vi "Graph MinMax X.vi"(8 "Fehler (Eingang, kein Fehler)":errorcluster, 10 "Max. Wert":dbl, 11 "Signalverlaufsdiagramm (Eingang)":refnum<vi>[](array[refnum])) -> (0 "Fehler (Ausgang)":errorcluster, 2 "Max. Wert out":dbl, 3 "Signalverlaufsdiagramm (Ausgang)":refnum<vi>[](array[refnum]))   [LabVIEW 2020, in "EPA 1065.lvlib" / "HovaCAL Interference verificaton.lvlib"]
uses:
  HovaCAL Interference verificaton.lvlib
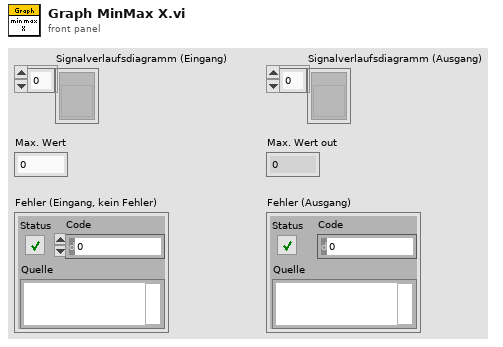
[diagram p1: front panel]
types:
  T1 = typedef "LVDateTimeRec.ctl" = cluster{"Sekundenbruchteil":dbl, "Sekunde":i32, "Minute":i32, "Stunde":i32, "Tag des Monats":i32, "Monat":i32, "Jahr":i32, "Wochentag":i32, "Tag des Jahres":i32, "DST":i32}
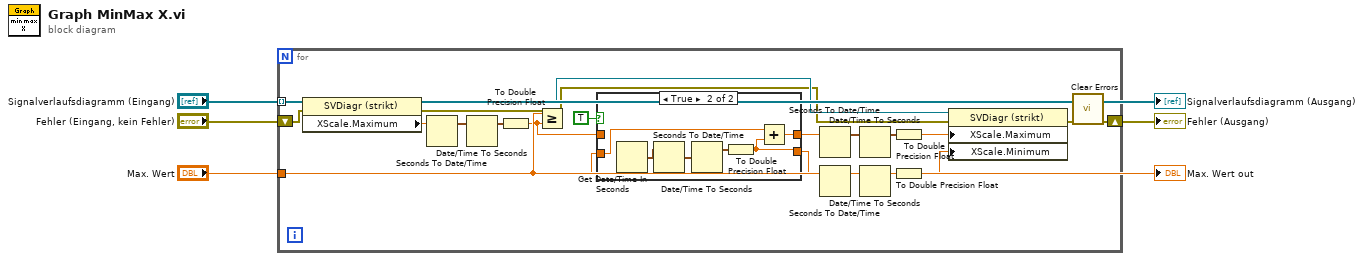
[diagram p0: block diagram]
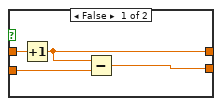
[diagram p2: hidden frame]
diagram:
  n1 = for {
    tunnel: "Max. Wert" -> [w23]
    tunnel: "Signalverlaufsdiagramm (Eingang)" -> [w22] mode=indexing
    shift-right: [w17] -> w2
    shift-left: "Fehler (Eingang, kein Fehler)" -> [w19]
    n2 = property on="Eigenschaftsknoten" class="SVDiagr (strikt)"(reference=w22, error in=w19) -> (reference out=w21:refnum<vi>, error out=w20:errorcluster, "XScale.Maximum"=w24:dbl)
    n3 = Seconds To Date/Time(time stamp (now)=w24) -> (date time rec=w16:T1)  [unwired: 1 in]
    n4 = Date/Time To Seconds(2:w16) -> (0:w14:timestamp)  [unwired: 1 in]
    n5 = To Double Precision Float(number=w14) -> (double precision float=w15:dbl)
    n6 = Greater Or Equal?(x=w23, y=w15) -> ()  [unwired: 1 out]
    n7 = case shown="True" TRUE ("x >= y?") {
      tunnel: w23 -> [w26 w34]
      tunnel: w15 -> [w28 _]
      tunnel: [w25 w30] -> w8
      tunnel: [w27 w29] -> w5
      frame False {
        n8 = Increment(x=w28) -> (x+1=w25:dbl)
        n9 = Subtract(x=w25, y=w26) -> (x-y=w27:dbl)
      }
      frame True {
        n10 = Get Date/Time In Seconds() -> (seconds since 1Jan1904=w32:timestamp)
        n11 = Seconds To Date/Time(time stamp (now)=w32) -> (date time rec=w31:T1)  [unwired: 1 in]
        n12 = Date/Time To Seconds(2:w31) -> (0:w33:timestamp)  [unwired: 1 in]
        n13 = To Double Precision Float(number=w33) -> (double precision float=w29:dbl)
        n14 = Add(x=w34, y=w29) -> (x+y=w30:dbl)
      }
    }
    n15 = Seconds To Date/Time(time stamp (now)=w8) -> (date time rec=w13:T1)  [unwired: 1 in]
    n16 = Seconds To Date/Time(time stamp (now)=w5) -> (date time rec=w9:T1)  [unwired: 1 in]
    n17 = Date/Time To Seconds(2:w13) -> (0:w12:timestamp)  [unwired: 1 in]
    n18 = Date/Time To Seconds(2:w9) -> (0:w10:timestamp)  [unwired: 1 in]
    n19 = To Double Precision Float(number=w12) -> (double precision float=w11:dbl)
    n20 = To Double Precision Float(number=w10) -> (double precision float=w7:dbl)
    n21 = property on="Eigenschaftsknoten" class="SVDiagr (strikt)"(reference=w21, error in=w20, "XScale.Maximum"=w11, "XScale.Minimum"=w7) -> (error out=w18:errorcluster)  [unwired: 1 out]
    n22 = call <vilib>:"Clear Errors.vi"("error in (no error)"=w18) -> ("error out"=w17:errorcluster)  [unwired: 5 in, 1 out]
  }
  "Fehler (Ausgang)" <- w2
  "Max. Wert out" <- "Max. Wert"
  "Signalverlaufsdiagramm (Ausgang)" <- "Signalverlaufsdiagramm (Eingang)"
